vi "INIT.vi"(8 "error in (no error)":errorcluster, 11 "DET_BUNCH in":refnum<class "Avantes_bunch.lvclass">) -> (0 "error out":errorcluster, 3 "DET_BUNCH out":refnum<class "Avantes_bunch.lvclass">)   [LabVIEW 2020, in "Avantes_bunch.lvclass"]
uses:
  Avantes_bunch.lvclass
  C:/Dev/TRANCON/Classes/Detector/Detector.lvclass
  Avantes_bunch.lvclass/Avantes_bunch.ctl
  Detector.lvclass/Detector.ctl
  Detector.lvclass
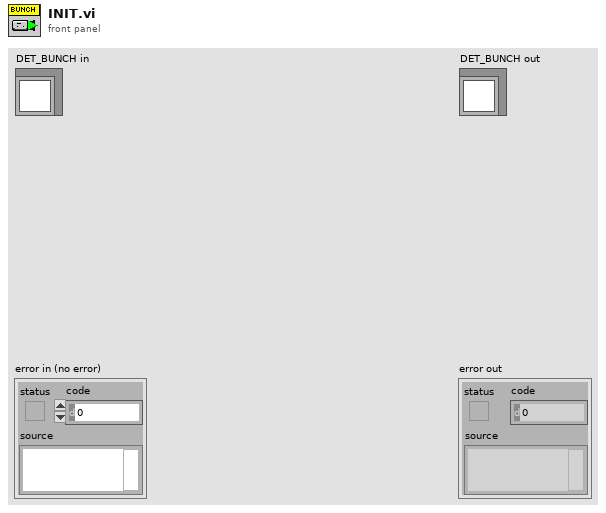
[diagram p1: front panel]
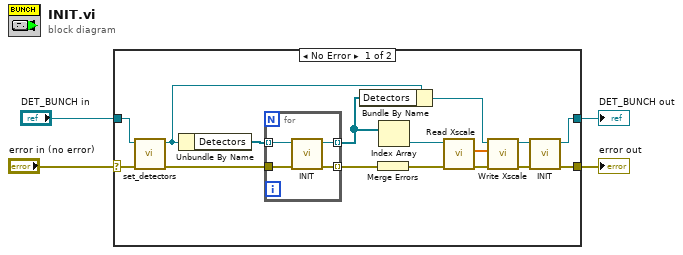
[diagram p0: block diagram]
diagram:
  n1 = case shown="No Error" "error in (no error)" {
    selector: "error in (no error)" -> [w17 w26]
    tunnel: [w7 w26] -> w3
    tunnel: [w8 w25] -> w2
    tunnel: "DET_BUNCH in" -> [w18 w25]
    frame No Error {
      n2 = call "set_detectors.vi"("error in (no error)"=w17, "DET_BUNCH in"=w18) -> ("error out"=w15:errorcluster, "DET_BUNCH out"=w16:refnum<class "Avantes_bunch.lvclass">)  [unwired: 8 in]
      n3 = Unbundle By Name(w16) -> ("Detectors"=w20:refnum<class "Detector.lvclass">[])
      n4 = for {
        tunnel: w20 -> [w24] mode=indexing
        tunnel: w15 -> [w23]
        tunnel: [w22] -> w19 mode=indexing
        tunnel: [w21] -> w13 mode=indexing
        n5 = call-dynamic "INIT.vi"("error in (no error)"=w23, "Detector in"=w24) -> ("error out"=w22:errorcluster, "Detector out"=w21:refnum<class "Detector.lvclass">)  [unwired: 8 in]
      }
      n6 = Bundle By Name(cluster=w16, "Detectors"=w13) -> (w6:refnum<class "Avantes_bunch.lvclass">)
      n7 = Merge Errors(w19) -> (w5:errorcluster)
      n8 = Index Array(array=w13) -> (element=w12:refnum<class "Detector.lvclass">)  [unwired: 1 in]
      n9 = call "Read Xscale.vi"("error in (no error)"=w5, "Detector en entrée"=w12) -> ("error out"=w11:errorcluster, "Xscale"=w14:dbl[])  [unwired: 7 in, 1 out]
      n10 = call "Write Xscale.vi"("error in (no error)"=w11, "Xscale"=w14, "Detector en entrée"=w6) -> ("error out"=w9:errorcluster, "Detector en sortie"=w10:refnum<class "Avantes_bunch.lvclass">)  [unwired: 7 in]
      n11 = call-parent "INIT.vi"("error in (no error)"=w9, "Detector in"=w10) -> ("error out"=w7:errorcluster, "Detector out"=w8:refnum<class "Avantes_bunch.lvclass">)  [unwired: 8 in]
    }
    frame Error {
    }
  }
  "error out" <- w3
  "DET_BUNCH out" <- w2
